vi "command_line_args.vi"(8 "error in (no error)":errorcluster, 10 "App.Args":string[](array[string]), 11 "Message Queues":T1) -> (0 "error out":errorcluster, 3 "2DArray":string[][](array[string]))   [LabVIEW 2013]
doc: "Receives the Command Line Arguments provided when the application was executed. The commands are decoded and translated to GUI sequence of GUI states for Main.vis"
uses:
  queues/que_all_message_queues.ctl
  queues/que_message_cluster.ctl
  type_def/general.ctl
  queues/que_enqueue_message_single.vi
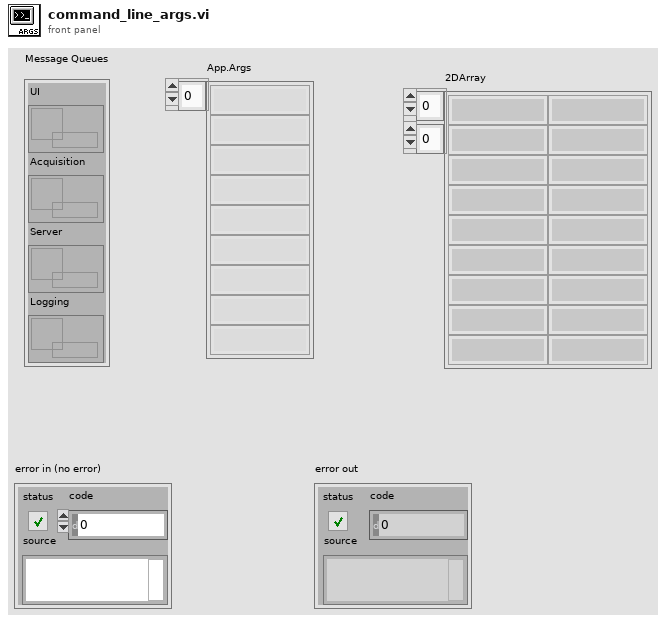
[diagram p1: front panel]
types:
  T1 = typedef "que_all_message_queues.ctl" = cluster{"UI":refnum<queue>, "Acquisition":refnum<queue>, "Server":refnum<queue>, "Logging":refnum<queue>}
  T2 = typedef "general.ctl" = cluster{"file_ext":string, "TCP port":i32, "#devices":i32, "log?":bool, "tcp?":bool, "language":string}
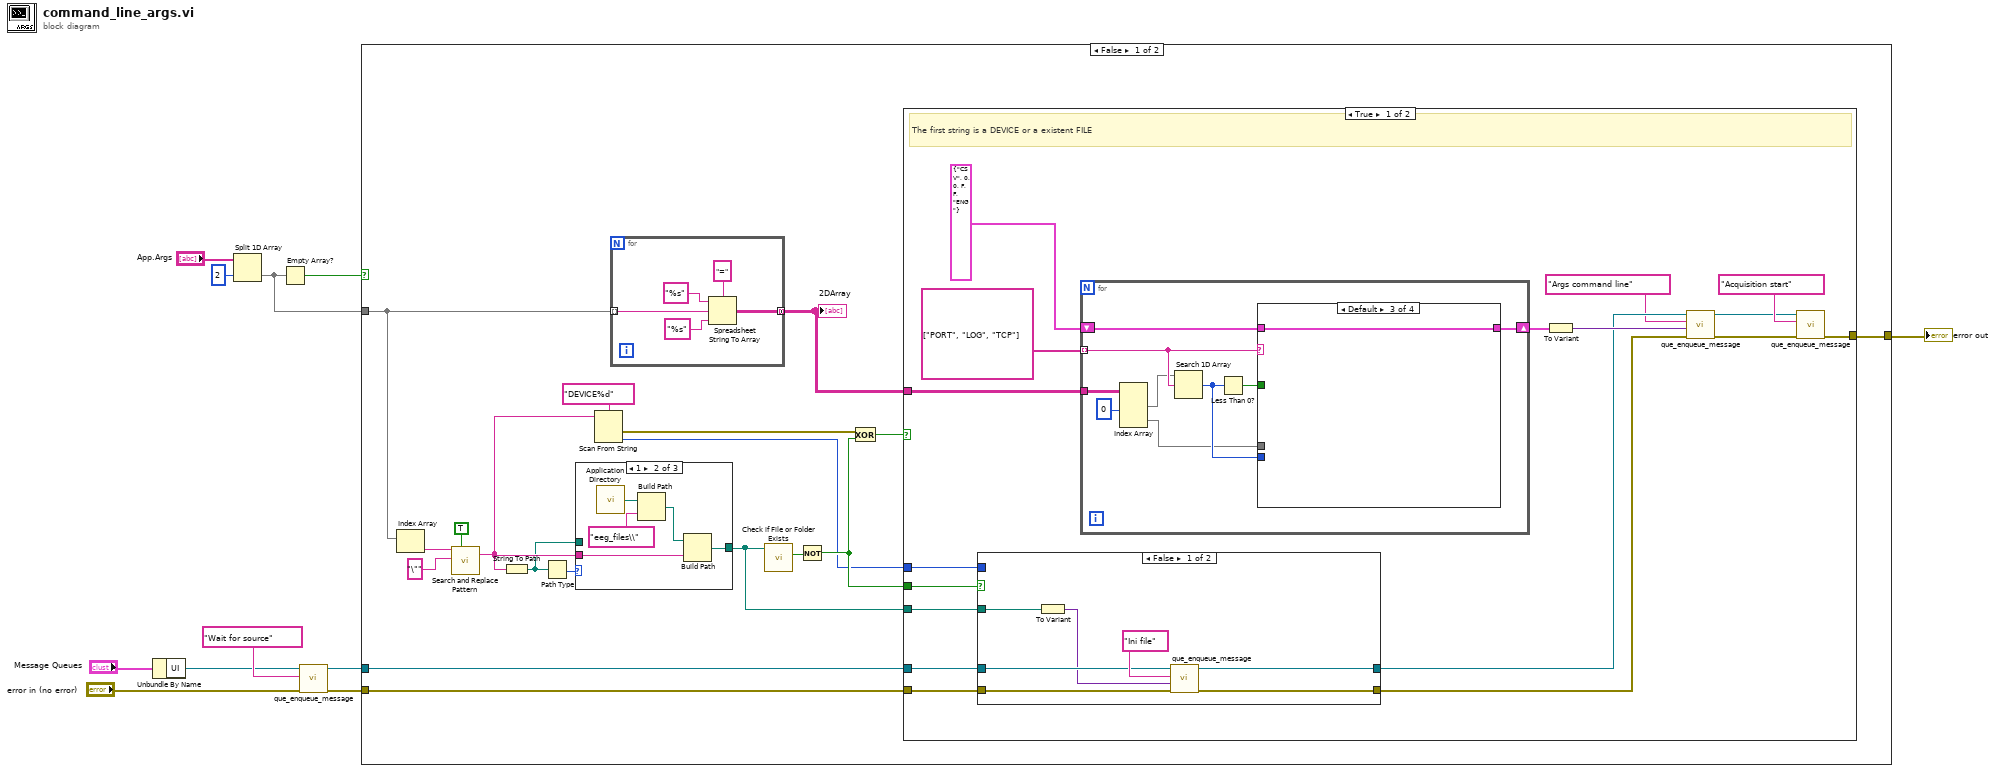
[diagram p0: block diagram]
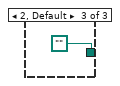
[diagram p3: hidden frame]
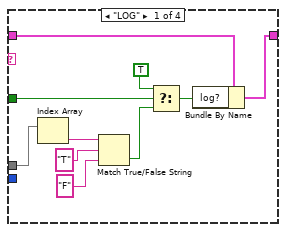
[diagram p4: hidden frame]
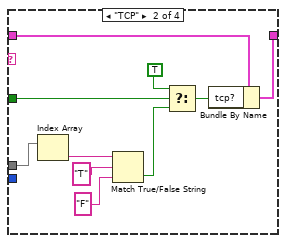
[diagram p5: hidden frame]
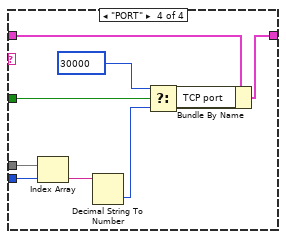
[diagram p6: hidden frame]
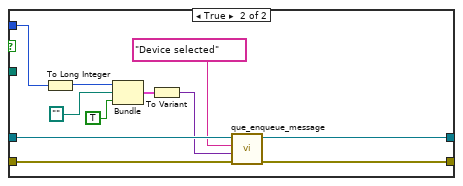
[diagram p7: hidden frame]
diagram:
  n1 = Unbundle By Name("Message Queues") -> ("UI"=w1:refnum<queue>)
  n2 = Split 1D Array(array="App.Args", index=2) -> (second subarray=w6:string[])  [unwired: 1 out]
  n3 = Empty Array?(array=w6) -> (empty?=w7:bool)
  n4 = call-poly "que_enqueue_message.vi"("error in (no error)"="error in (no error)", "Message"="Wait for source", "Message Queue"=w1) -> ("error out"=w3:errorcluster, "dup Message Queue"=w4:refnum<queue>)  [unwired: 7 in]
  n5 = case shown="False" w7 {
    tunnel: [w29 w117] -> w10
    tunnel: w3 -> [w12 w117]
    tunnel: w4 -> [w13 _]
    tunnel: w6 -> [w14 _]
    frame False {
      n6 = Index Array(array=w14) -> (element=w27:string)  [unwired: 1 in]
      n7 = call <vilib>:"Search and Replace Pattern.vi"("string"=w27, "regular expression (\"\")"="\"" ("regular expression (\"\")"), "replace all? (F)"=TRUE) -> ("result string"=w23:string)  [unwired: 2 in, 1 out]
      n8 = String To Path(string=w23) -> (path=w22:path)
      n9 = Path Type(1:w22) -> (0:w24:i16)
      n10 = case shown="1" w24 {
        tunnel: w23 -> [_ w35 _]
        tunnel: [w30 w31 path ""] -> w17
        tunnel: w22 -> [w30 _ _]
        frame 0 {
        }
        frame 1 {
          n11 = call <vilib>:"Application Directory.vi"() -> ("Application Directory"=w34:path)
          n12 = Build Path(base path=w34, name or relative path="eeg_files\\") -> (appended path=w32:path)
          n13 = Build Path(base path=w32, name or relative path=w35) -> (appended path=w31:path)
        }
        frame 2, Default {
        }
      }
      n14 = Scan From String(format string="DEVICE%d", input string=w23) -> (error out=w21:errorcluster, output 1=w16:i32)  [unwired: 3 in, 2 out]
      n15 = for {
        tunnel: w14 -> [w38] mode=indexing
        tunnel: [w37] -> w15 mode=concatenating
        n16 = Spreadsheet String To Array(delimiter (Tab)="=", format string="%s", spreadsheet string=w38, array type (2D Dbl)="%s" ("format string")) -> (array=w37:string[][])
      }
      "2DArray" <- w15
      n17 = call <vilib>:"Check if File or Folder Exists.vi"("path"=w17) -> ("file or folder exists?"=w20:bool)  [unwired: 8 in, 2 out]
      n18 = Not(x=w20) -> (.not. x?=w18:bool)
      n19 = Exclusive Or(1:w18, 2:w21) -> (0:w19:bool)
      n20 = case shown="True" w19 {
        tunnel: w12 -> [w43 w116]
        tunnel: [w49 w116] -> w29
        tunnel: w15 -> [w48 _]
        tunnel: w18 -> [w47 _]
        tunnel: w17 -> [w46 _]
        tunnel: w16 -> [w45 _]
        tunnel: w13 -> [w44 _]
        frame True {
          # "The first string is a DEVICE or a existent FILE"
          n21 = case shown="False" w47 {
            tunnel: w44 -> [w103 w115]
            tunnel: [w100 w109] -> w56
            tunnel: [w99 w108] -> w55
            tunnel: w43 -> [w98 w107]
            tunnel: w46 -> [w101 _]
            tunnel: w45 -> [_ w106]
            frame False {
              n22 = To Variant(anything=w101) -> (Variant=w102:variant)
              n23 = call-poly "que_enqueue_message.vi"("error in (no error)"=w98, "Message Data"=w102, "Message"="Ini file", "Message Queue"=w103) -> ("error out"=w99:errorcluster, "dup Message Queue"=w100:refnum<queue>)  [unwired: 6 in]
            }
            frame True {
              n24 = To Long Integer(number=w106) -> (32bit integer=w113:i32)
              n25 = Bundle(w113, path "", TRUE) -> (w112:cluster{i32, path, bool})  [unwired: 1 in]
              n26 = To Variant(anything=w112) -> (Variant=w111:variant)
              n27 = call-poly "que_enqueue_message.vi"("error in (no error)"=w107, "Message Data"=w111, "Message"="Device selected", "Message Queue"=w115) -> ("error out"=w108:errorcluster, "dup Message Queue"=w109:refnum<queue>)  [unwired: 6 in]
            }
          }
          n28 = for {
            tunnel: string[] ["PORT", "LOG", "TCP"] -> [w64] mode=indexing
            shift-right: [w66] -> w50
            shift-left: T2 {"file_ext"="CSV", "TCP port"=0, "#devices"=0, "log?"=FALSE, "tcp?"=FALSE, "language"="ENG"} ("general") -> [w65]
            tunnel: w48 -> [w61]
            n29 = Index Array(array=w61, index (col) #1=0 ("disabled index (col)")) -> (element #1=w60:string[], element #2=w59:string[])  [unwired: 3 in]
            n30 = Search 1D Array(1D array=w60, element=w64) -> (index of element=w67:i32)  [unwired: 1 in]
            n31 = Less Than 0?(x=w67) -> (x < 0?=w63:bool)
            n32 = case shown="Default" w64 {
              tunnel: w67 -> [_ _ _ w93]
              tunnel: [w76 w86 w88 w96] -> w66
              tunnel: w65 -> [w77 w87 w88 w97]
              tunnel: w63 -> [w75 w85 _ w95]
              tunnel: w59 -> [w73 w83 _ w90]
              frame "LOG" {
                n33 = Index Array(array=w73) -> (element=w72:string)  [unwired: 1 in]
                n34 = Match True/False String(2:"F" ("false string"), 3:"T" ("true string"), 4:w72) -> (0:w69:bool)  [unwired: 1 out]
                n35 = Select(t=TRUE, s=w75, f=w69) -> (s? t:f=w68:bool)
                n36 = Bundle By Name(cluster=w77, "log?"=w68) -> (w76:T2)
              }
              frame "TCP" {
                n37 = Index Array(array=w83) -> (element=w82:string)  [unwired: 1 in]
                n38 = Match True/False String(2:"F" ("false string"), 3:"T" ("true string"), 4:w82) -> (0:w79:bool)  [unwired: 1 out]
                n39 = Select(t=TRUE, s=w85, f=w79) -> (s? t:f=w78:bool)
                n40 = Bundle By Name(cluster=w87, "tcp?"=w78) -> (w86:T2)
              }
              frame Default {
              }
              frame "PORT" {
                n41 = Index Array(array=w90, index=w93) -> (element=w89:string)
                n42 = Decimal String To Number(string=w89) -> (number=w92:i32)  [unwired: 2 in, 1 out]
                n43 = Select(t=30000 ("general.port"), s=w95, f=w92) -> (s? t:f=w91:i32)
                n44 = Bundle By Name(cluster=w97, "TCP port"=w91) -> (w96:T2)
              }
            }
          }
          n45 = To Variant(anything=w50) -> (Variant=w57:variant)
          n46 = call-poly "que_enqueue_message.vi"("error in (no error)"=w55, "Message Data"=w57, "Message"="Args command line", "Message Queue"=w56) -> ("error out"=w51:errorcluster, "dup Message Queue"=w52:refnum<queue>)  [unwired: 6 in]
          n47 = call-poly "que_enqueue_message.vi"("error in (no error)"=w51, "Message"="Acquisition start", "Message Queue"=w52) -> ("error out"=w49:errorcluster)  [unwired: 7 in, 1 out]
        }
        frame False {
          # "The first string in not a DEVICE nor a existent FILE"
        }
      }
    }
    frame True {
    }
  }
  "error out" <- w10
